vi "Get Reference Timestamp.vi"(11 "PCAN Base Strategy in":refnum<class "PCAN Base Strategy.lvclass">) -> (2 "Reference Timestamp":timestamp format="%<%x %.3X>T", 3 "PCAN Base Strategy out":refnum<class "PCAN Base Strategy.lvclass">)   [LabVIEW 2024, in "PCAN Base Strategy.lvclass"]
uses:
  PCAN Base Strategy.lvclass
  PCAN Base Strategy.lvclass/PCAN Base Strategy.ctl
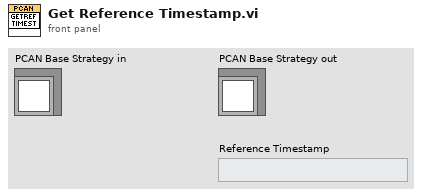
[diagram p1: front panel]
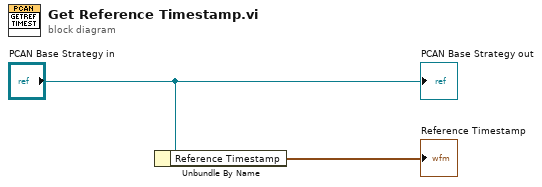
[diagram p0: block diagram]
diagram:
  n1 = Unbundle By Name("PCAN Base Strategy in") -> ("Reference Timestamp"=→"Reference Timestamp":timestamp)
  "PCAN Base Strategy out" <- "PCAN Base Strategy in"
